vi "API_Sync CMD DoSomething.vi"(8 "error in (no error)":errorcluster, 9 "vData":variant, 11 "DLP2 in":refnum<class "DLP2.lvclass">) -> (0 "error out":errorcluster, 3 "DLP2 out":refnum<class "DLP2.lvclass">)   [LabVIEW 2022 SP3, in "DLP2.lvclass"]
doc: "Developed by Kevin Thompson\nkevin@thompsonengineering.net\n\nCopyright 2018\nThompson Engineering, LLC"
uses:
  DLP2.lvclass
  DataTypes/AsynCmd_Temp01--enum.ctl
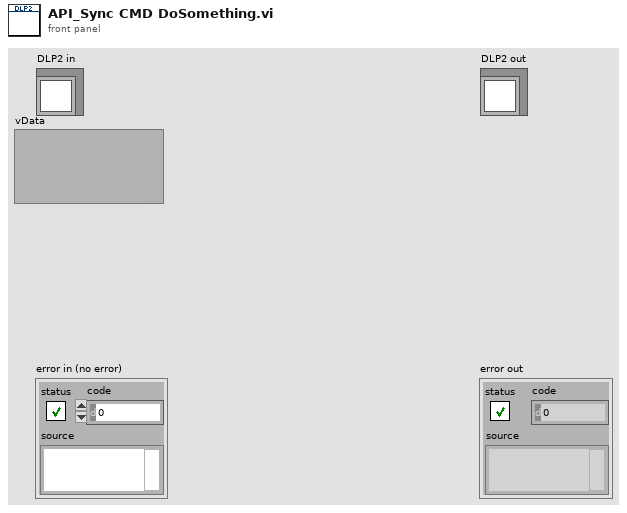
[diagram p1: front panel]
types:
  T1 = typedef "DLP2.lvclass/AsynCmd_Temp01--enum.ctl" = enum16{"LoadTiffImage"}
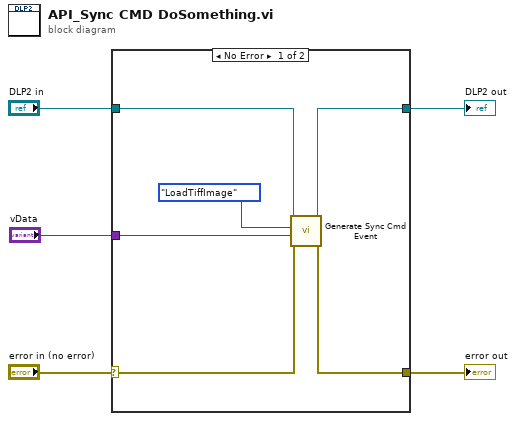
[diagram p0: block diagram]
diagram:
  n1 = case shown="No Error" "error in (no error)" {
    selector: "error in (no error)" -> [w9 w13]
    tunnel: [w8 w13] -> w4
    tunnel: [w10 w12] -> w2
    tunnel: "DLP2 in" -> [w11 w12]
    tunnel: "vData" -> [w6 _]
    frame No Error {
      n2 = call "Generate Sync Cmd Event.vi"("error in (no error)"=w9, "vData"=w6, "AsyncCmd"=AsynCmd_Temp01--enum."LoadTiffImage", "DLP2 in"=w11) -> ("error out"=w8:errorcluster, "DLP2 out"=w10:refnum<class "DLP2.lvclass">)  [unwired: 5 in, 1 out]
    }
    frame Error {
    }
  }
  "error out" <- w4
  "DLP2 out" <- w2
